vi "Reset Graph Axes.vi"(8 "error in (no error)":errorcluster, 10 "Measurement UI Controls":T14, 11 "Settings":T1) -> (0 "error out":errorcluster, 3 "Settings out":T1)   [LabVIEW 2021]
doc: "Make both Y Axes visible and set their ranges."
uses:
  Settings/Settings.ctl
  Acquisition/Hardware Configuration.ctl
  Acquisition/Channel Settings.ctl
  Acquisition/IO Device.ctl
  Acquisition/Sensor Type.ctl
  Interval Timer/Repeat Interval.ctl
  Interval Timer/Interval Length.ctl
  Interval Timer/Interval Token.ctl
  Acquisition/IO API.ctl
  Logging/Logging Configuration.ctl
  Logging/Logging Mode.ctl
  Diagnostics/Diagnostics Configuration.ctl
  controls/Graph Settings.ctl
  controls/UI Data.ctl
  Acquisition/Acquisition.lvlib
  Interval Timer/Interval Timer.lvlib
  Logging/Logging.lvlib
  Diagnostics/Diagnostics.lvlib
  Settings/Settings.lvlib
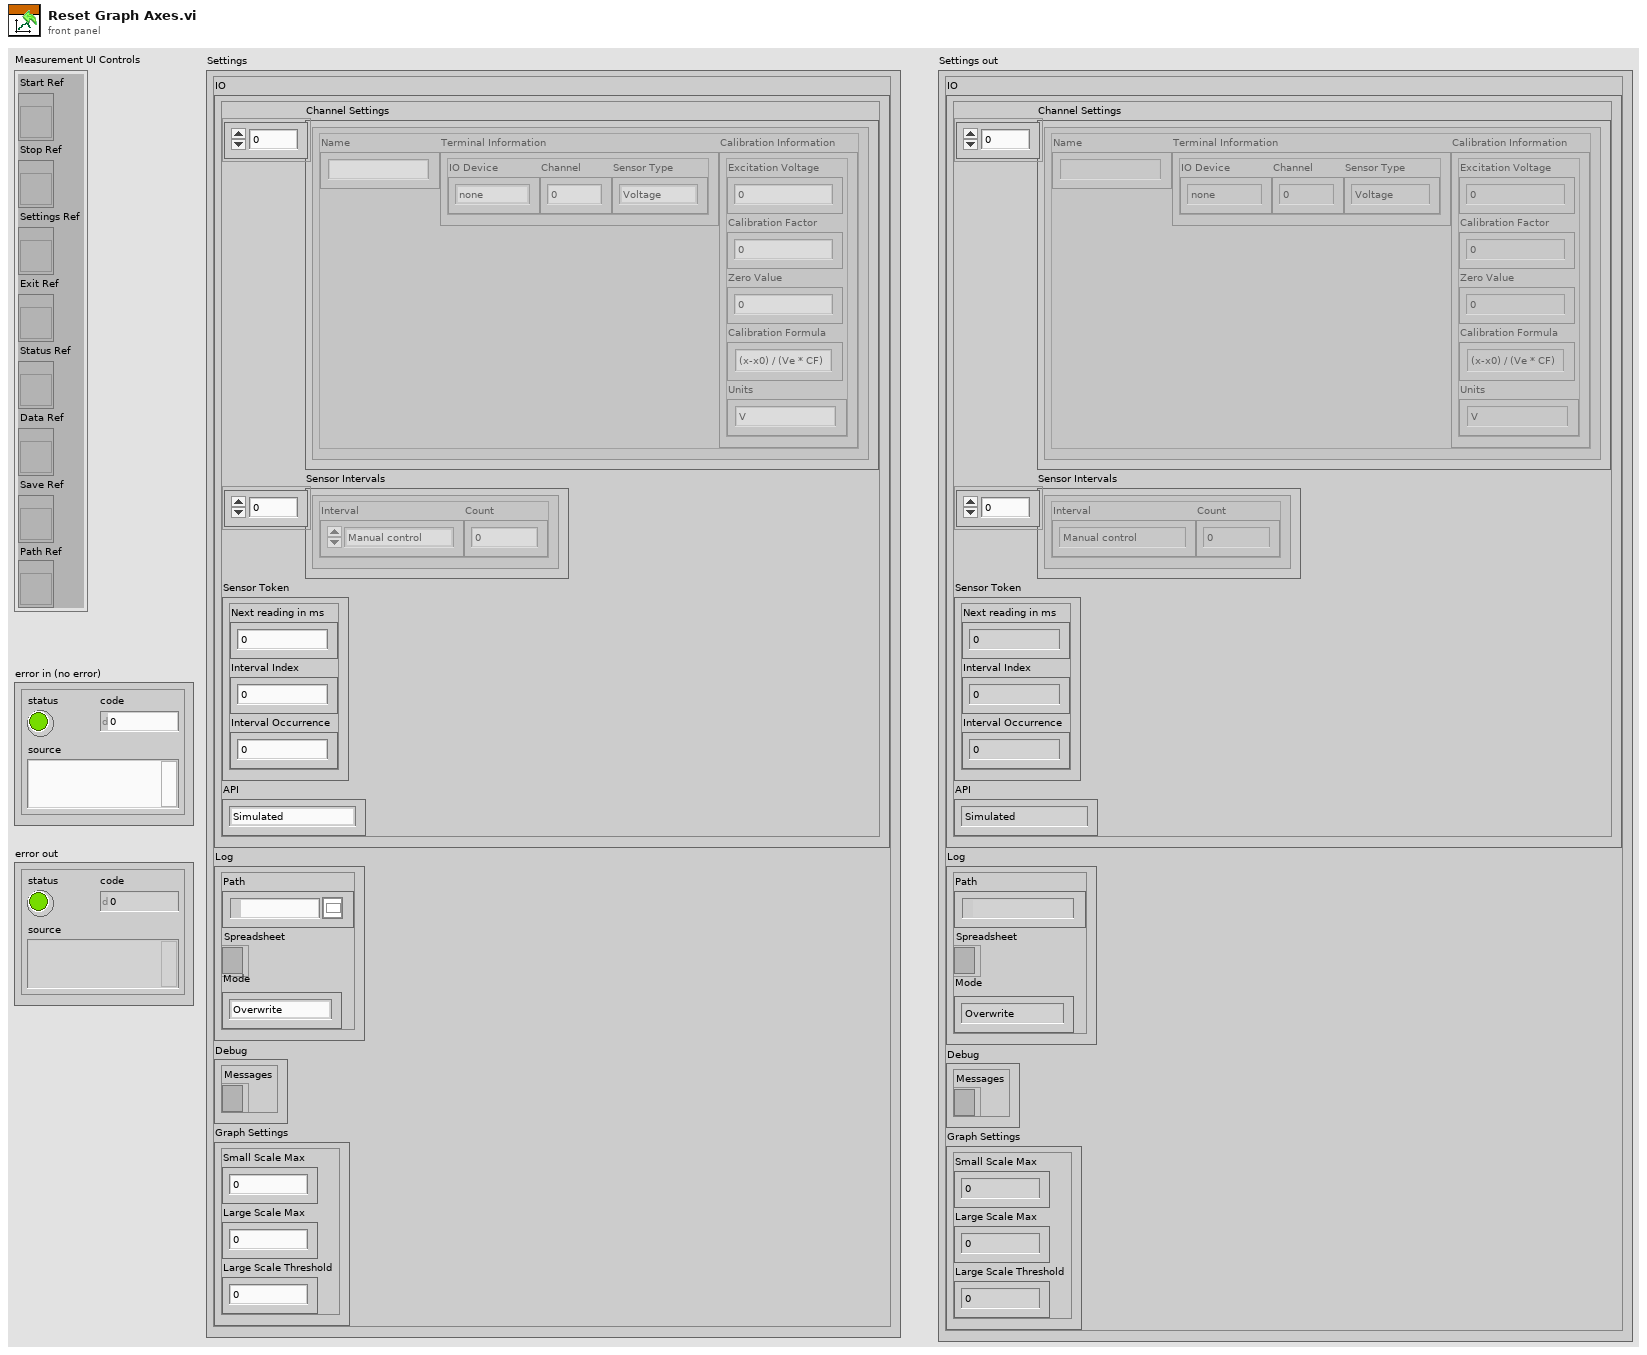
[diagram p1: front panel]
types:
  T1 = typedef "Settings.lvlib/Settings.ctl" = cluster{"IO":T2, "Log":T10, "Debug":T12, "Graph Settings":T13}
  T2 = typedef "Acquisition.lvlib/Hardware Configuration.ctl" = cluster{"Channel Settings":T3[], "Sensor Intervals":T6[], "Sensor Token":T8, "API":T9}
  T3 = typedef "Acquisition.lvlib/Channel Settings.ctl" = cluster{"Name":string, "Terminal Information":cluster{"IO Device":T4, "Channel":i32, "Sensor Type":T5}, "Calibration Information":cluster{"Excitation Voltage":dbl, "Calibration Factor":dbl, "Zero Value":dbl, "Calibration Formula":string, "Units":string}}
  T4 = typedef "Acquisition.lvlib/IO Device.ctl" = enum16{"none", "9219", "9401"}
  T5 = typedef "Acquisition.lvlib/Sensor Type.ctl" = enum16{"Voltage", "Load", "Pressure", "Encoder"}
  T6 = typedef "Interval Timer.lvlib/Repeat Interval.ctl" = cluster{"Interval":T7, "Count":i32}
  T7 = typedef "Interval Timer.lvlib/Interval Length.ctl" = enum16{"Manual control", "1 second", "10 seconds", "30 seconds", "60 seconds", "600 seconds", "1200 seconds", "3600 seconds"}
  T8 = typedef "Interval Timer.lvlib/Interval Token.ctl" = cluster{"Next reading in ms":u32, "Interval Index":i32, "Interval Occurrence":i32}
  T9 = typedef "Acquisition.lvlib/IO API.ctl" = enum16{"Simulated", "DAQmx"}
  T10 = typedef "Logging.lvlib/Logging Configuration.ctl" = cluster{"Path":path, "Spreadsheet":refnum<file>, "Mode":T11}
  T11 = typedef "Logging.lvlib/Logging Mode.ctl" = enum16{"Overwrite", "Append", "Create New"}
  T12 = typedef "Diagnostics.lvlib/Diagnostics Configuration.ctl" = cluster{"Messages":refnum<file>}
  T13 = typedef "Graph Settings.ctl" = cluster{"Small Scale Max":dbl, "Large Scale Max":dbl, "Large Scale Threshold":dbl}
  T14 = typedef "UI Data.ctl" = cluster{"Start Ref":refnum<vi>, "Stop Ref":refnum<vi>, "Settings Ref":refnum<vi>, "Exit Ref":refnum<vi>, "Status Ref":refnum<vi>, "Data Ref":refnum<vi>, "Save Ref":refnum<vi>, "Path Ref":refnum<vi>}
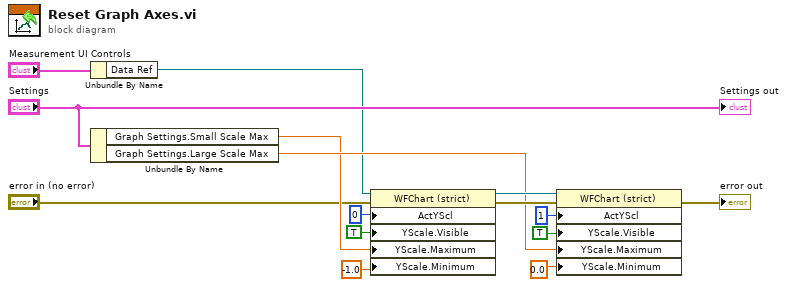
[diagram p0: block diagram]
diagram:
  n1 = Unbundle By Name("Measurement UI Controls") -> ("Data Ref"=w2:refnum<vi>)
  n2 = Unbundle By Name("Settings") -> ("Graph Settings.Small Scale Max"=w4:dbl, "Graph Settings.Large Scale Max"=w5:dbl)
  n3 = property class="WFChart (strict)"(reference=w2, error in="error in (no error)", "ActYScl"=0 ("Active Y Scale"), "YScale.Visible"=TRUE ("Y Scale.Visible"), "YScale.Maximum"=w4, "YScale.Minimum"=-1.0 ("Y Scale.Range:Maximum")) -> (reference out=w9:refnum<vi>, error out=w10:errorcluster)
  n4 = property class="WFChart (strict)"(reference=w9, error in=w10, "ActYScl"=1 ("Active Y Scale"), "YScale.Visible"=TRUE ("Y Scale.Visible"), "YScale.Maximum"=w5, "YScale.Minimum"=0.0 ("Y Scale.Range:Maximum")) -> (error out=→"error out":errorcluster)  [unwired: 1 out]
  "Settings out" <- "Settings"
